vi "SimultaneusWaveformStart.vi"(5 "Ch5Start":bool, 6 "Ch6Start":bool, 7 "Ch4Start":bool, 8 "Ch3Start":bool, 9 "Ch2Start":bool, 10 "Ch1Start":bool, 11 "Handle":u32) -> (3 "FT_Status":u32(ring) items=["FT_OK", "FT_INVALID_HANDLE", "FT_DEVICE_NOT_FOUND", "FT_DEVICE_NOT_OPENED", "FT_IO_ERROR", "FT_INSUFFICIENT_RESOURCES", "FT_INVALID_PARAMETER", "FT_INVALID_BAUD_RATE", "FT_DEVICE_NOT_OPENED_FOR_ERASE", "FT_DEVICE_NOT_OPENED_FOR_WRITE", "FT_FAILED_TO_WRITE_DEVICE", "FT_EEPROM_READ_FAILED", "FT_EEPROM_WRITE_FAILED", "FT_EEPROM_ERASE_FAILED", "FT_EEPROM_NOT_PRESENT", "FT_EEPROM_NOT_PROGRAMMED", "FT_INVALID_ARGS", "FT_NOT_SUPPORTED", "FT_OTHER_ERROR"])   [LabVIEW 2013]
panel:
  out "Bytes Written":u32
  out "Start Array":u8[](array[numeric])
  out "Enable Array":u8[](array[numeric])
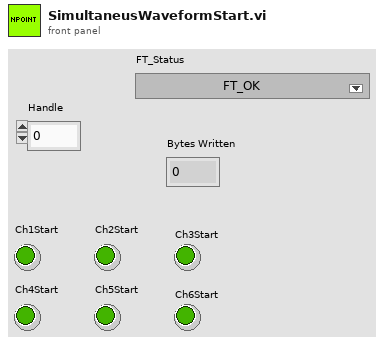
[diagram p1: front panel]
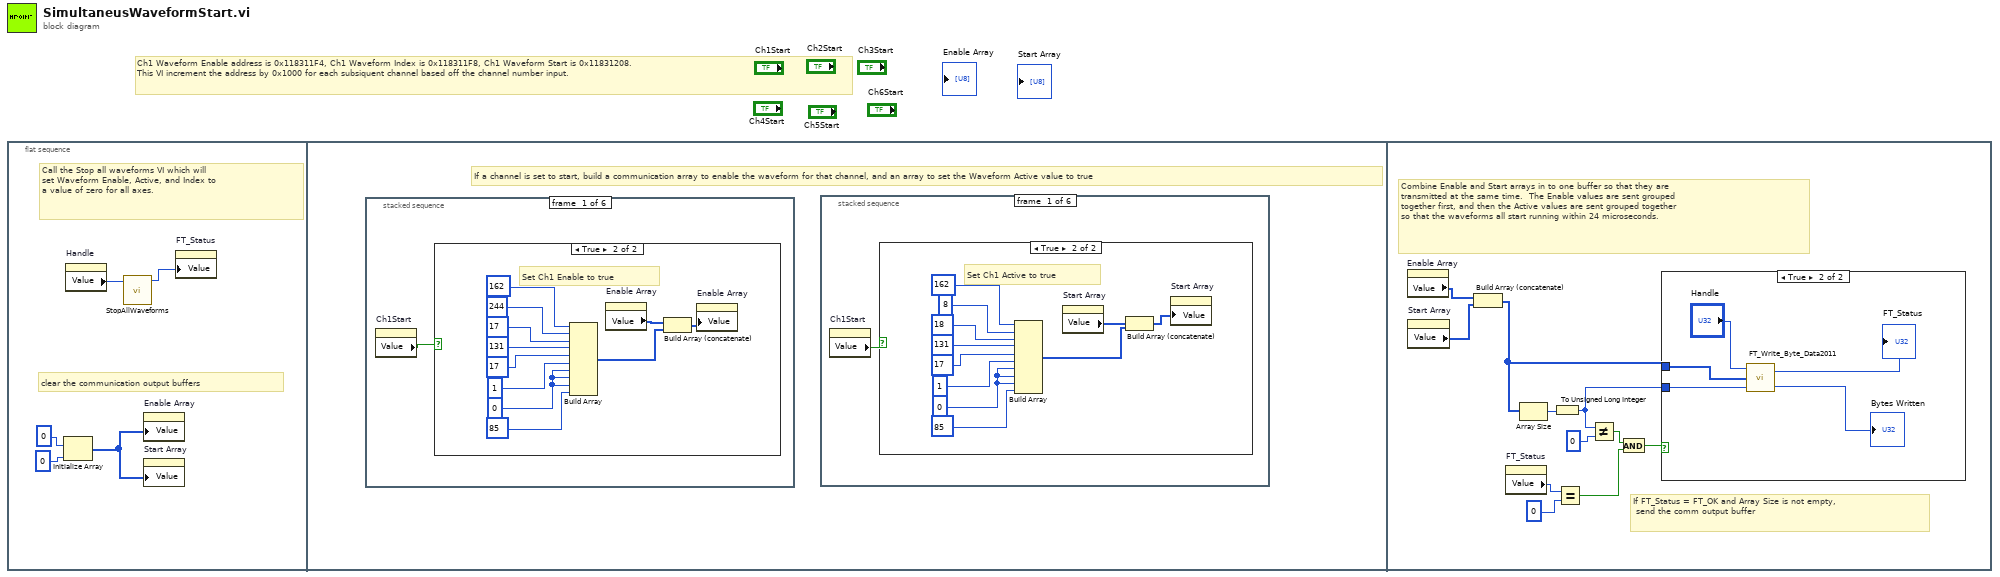
[diagram p0: block diagram]
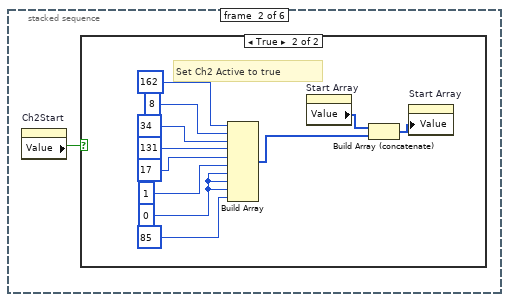
[diagram p3: hidden frame]
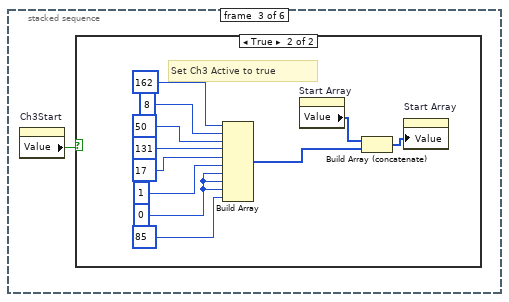
[diagram p5: hidden frame]
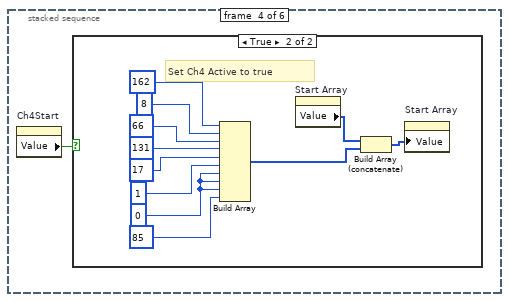
[diagram p7: hidden frame]
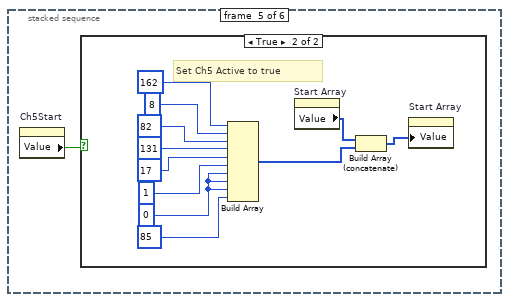
[diagram p9: hidden frame]
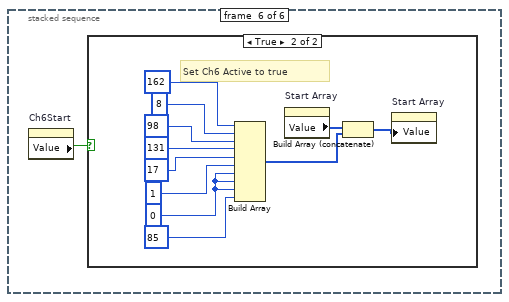
[diagram p11: hidden frame]
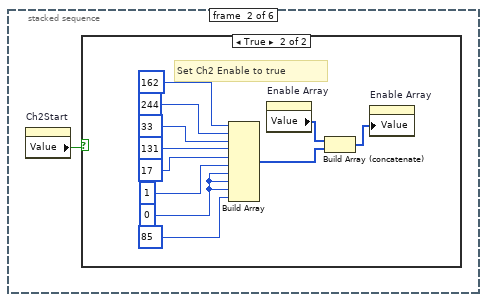
[diagram p14: hidden frame]
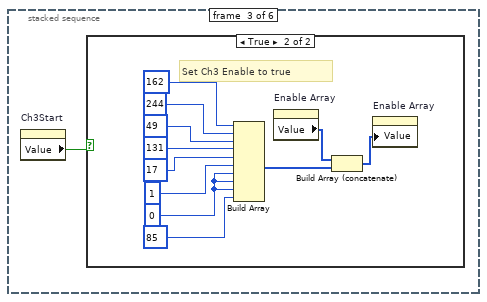
[diagram p16: hidden frame]
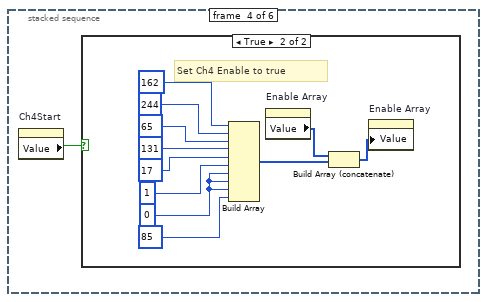
[diagram p18: hidden frame]
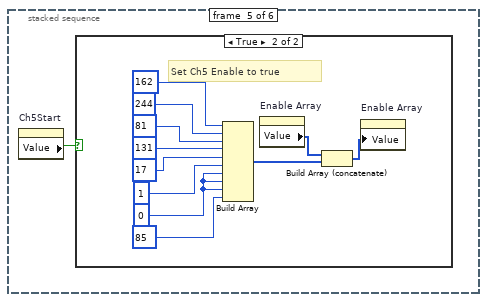
[diagram p20: hidden frame]
diagram:
  # "Ch1 Waveform Enable address is 0x118311F4, Ch1 Waveform Index is 0x118311F8, Ch1 Waveform Start is 0x11831208.\nThis VI increment the address by 0x1000 for each subsiquent channel based off the channel number input."
  n1 = flat-sequence {
    frame #0 {
      # "clear the communication output buffers"
      # "Call the Stop all waveforms VI which will\nset Waveform Enable, Active, and Index to \na value of zero for all axes."
      n2 = Initialize Array(u8 0, 0 ("dimension size")) -> (w1:u8[])
      n3 = property on="Handle" class="DigNum (strict)"() -> ("Value"=w5:u32)  [unwired: 2 in, 2 out]
      n4 = call "StopAllWaveforms.vi"("Handle"=w5) -> ("FT_Status"=w4:u32)  [unwired: 10 in]
      n5 = property on="Enable Array" class="Arr (strict)"("Value"=w1) -> ()  [unwired: 2 in, 2 out]
      n6 = property on="Start Array" class="Arr (strict)"("Value"=w1) -> ()  [unwired: 2 in, 2 out]
      n7 = property on="FT_Status" class="Ring (strict)"("Value"=w4) -> ()  [unwired: 2 in, 2 out]
    }
    frame #1 {
      # "If a channel is set to start, build a communication array to enable the waveform for that channel, and an array to set the Waveform Active value to true"
      n8 = stacked-sequence {
        frame #0 {
          n9 = property on="Ch1Start" class="Bool (strict)"() -> ("Value"=w78:bool)  [unwired: 2 in, 2 out]
          n10 = case shown="True" w78 {
            frame False {
            }
            frame True {
              w83 = u8 0 ("element")
              # "Set Ch1 Enable to true"
              n11 = Build Array(u8 162 ("element"), u8 244 ("element"), u8 17 ("element"), u8 131 ("element"), u8 17 ("element"), u8 1 ("element"), w83, w83, w83, u8 85 ("element")) -> (w80:u8[])
              n12 = property on="Enable Array" class="Arr (strict)"() -> ("Value"=w81:u8[])  [unwired: 2 in, 2 out]
              n13 = Build Array (concatenate)(w81, w80) -> (w79:u8[])
              n14 = property on="Enable Array" class="Arr (strict)"("Value"=w79) -> ()  [unwired: 2 in, 2 out]
            }
          }
        }
        frame #1 {
          n15 = property on="Ch2Start" class="Bool (strict)"() -> ("Value"=w90:bool)  [unwired: 2 in, 2 out]
          n16 = case shown="True" w90 {
            frame False {
            }
            frame True {
              w95 = u8 0 ("element")
              # "Set Ch2 Enable to true"
              n17 = Build Array(u8 162 ("element"), u8 244 ("element"), u8 33 ("element"), u8 131 ("element"), u8 17 ("element"), u8 1 ("element"), w95, w95, w95, u8 85 ("element")) -> (w92:u8[])
              n18 = property on="Enable Array" class="Arr (strict)"() -> ("Value"=w93:u8[])  [unwired: 2 in, 2 out]
              n19 = Build Array (concatenate)(w93, w92) -> (w91:u8[])
              n20 = property on="Enable Array" class="Arr (strict)"("Value"=w91) -> ()  [unwired: 2 in, 2 out]
            }
          }
        }
        frame #2 {
          n21 = property on="Ch3Start" class="Bool (strict)"() -> ("Value"=w102:bool)  [unwired: 2 in, 2 out]
          n22 = case shown="True" w102 {
            frame False {
            }
            frame True {
              w107 = u8 0 ("element")
              # "Set Ch3 Enable to true"
              n23 = Build Array(u8 162 ("element"), u8 244 ("element"), u8 49 ("element"), u8 131 ("element"), u8 17 ("element"), u8 1 ("element"), w107, w107, w107, u8 85 ("element")) -> (w104:u8[])
              n24 = property on="Enable Array" class="Arr (strict)"() -> ("Value"=w105:u8[])  [unwired: 2 in, 2 out]
              n25 = Build Array (concatenate)(w105, w104) -> (w103:u8[])
              n26 = property on="Enable Array" class="Arr (strict)"("Value"=w103) -> ()  [unwired: 2 in, 2 out]
            }
          }
        }
        frame #3 {
          n27 = property on="Ch4Start" class="Bool (strict)"() -> ("Value"=w114:bool)  [unwired: 2 in, 2 out]
          n28 = case shown="True" w114 {
            frame False {
            }
            frame True {
              w119 = u8 0 ("element")
              # "Set Ch4 Enable to true"
              n29 = Build Array(u8 162 ("element"), u8 244 ("element"), u8 65 ("element"), u8 131 ("element"), u8 17 ("element"), u8 1 ("element"), w119, w119, w119, u8 85 ("element")) -> (w116:u8[])
              n30 = property on="Enable Array" class="Arr (strict)"() -> ("Value"=w117:u8[])  [unwired: 2 in, 2 out]
              n31 = Build Array (concatenate)(w117, w116) -> (w115:u8[])
              n32 = property on="Enable Array" class="Arr (strict)"("Value"=w115) -> ()  [unwired: 2 in, 2 out]
            }
          }
        }
        frame #4 {
          n33 = property on="Ch5Start" class="Bool (strict)"() -> ("Value"=w126:bool)  [unwired: 2 in, 2 out]
          n34 = case shown="True" w126 {
            frame False {
            }
            frame True {
              w131 = u8 0 ("element")
              # "Set Ch5 Enable to true"
              n35 = Build Array(u8 162 ("element"), u8 244 ("element"), u8 81 ("element"), u8 131 ("element"), u8 17 ("element"), u8 1 ("element"), w131, w131, w131, u8 85 ("element")) -> (w128:u8[])
              n36 = property on="Enable Array" class="Arr (strict)"() -> ("Value"=w129:u8[])  [unwired: 2 in, 2 out]
              n37 = Build Array (concatenate)(w129, w128) -> (w127:u8[])
              n38 = property on="Enable Array" class="Arr (strict)"("Value"=w127) -> ()  [unwired: 2 in, 2 out]
            }
          }
        }
        frame #5 {
          n39 = property on="Ch6Start" class="Bool (strict)"() -> ("Value"=w138:bool)  [unwired: 2 in, 2 out]
          n40 = case shown="True" w138 {
            frame False {
            }
            frame True {
              w143 = u8 0 ("element")
              # "Set Ch6 Enable to true"
              n41 = Build Array(u8 162 ("element"), u8 244 ("element"), u8 97 ("element"), u8 131 ("element"), u8 17 ("element"), u8 1 ("element"), w143, w143, w143, u8 85 ("element")) -> (w140:u8[])
              n42 = property on="Enable Array" class="Arr (strict)"() -> ("Value"=w141:u8[])  [unwired: 2 in, 2 out]
              n43 = Build Array (concatenate)(w141, w140) -> (w139:u8[])
              n44 = property on="Enable Array" class="Arr (strict)"("Value"=w139) -> ()  [unwired: 2 in, 2 out]
            }
          }
        }
      }
      n45 = stacked-sequence {
        frame #0 {
          n46 = property on="Ch1Start" class="Bool (strict)"() -> ("Value"=w6:bool)  [unwired: 2 in, 2 out]
          n47 = case shown="True" w6 {
            frame False {
            }
            frame True {
              w11 = u8 0 ("element")
              # "Set Ch1 Active to true"
              n48 = Build Array(u8 162 ("element"), u8 8 ("element"), u8 18 ("element"), u8 131 ("element"), u8 17 ("element"), u8 1 ("element"), w11, w11, w11, u8 85 ("element")) -> (w8:u8[])
              n49 = property on="Start Array" class="Arr (strict)"() -> ("Value"=w9:u8[])  [unwired: 2 in, 2 out]
              n50 = Build Array (concatenate)(w9, w8) -> (w7:u8[])
              n51 = property on="Start Array" class="Arr (strict)"("Value"=w7) -> ()  [unwired: 2 in, 2 out]
            }
          }
        }
        frame #1 {
          n52 = property on="Ch2Start" class="Bool (strict)"() -> ("Value"=w18:bool)  [unwired: 2 in, 2 out]
          n53 = case shown="True" w18 {
            frame False {
            }
            frame True {
              w23 = u8 0 ("element")
              # "Set Ch2 Active to true"
              n54 = Build Array(u8 162 ("element"), u8 8 ("element"), u8 34 ("element"), u8 131 ("element"), u8 17 ("element"), u8 1 ("element"), w23, w23, w23, u8 85 ("element")) -> (w20:u8[])
              n55 = property on="Start Array" class="Arr (strict)"() -> ("Value"=w21:u8[])  [unwired: 2 in, 2 out]
              n56 = Build Array (concatenate)(w21, w20) -> (w19:u8[])
              n57 = property on="Start Array" class="Arr (strict)"("Value"=w19) -> ()  [unwired: 2 in, 2 out]
            }
          }
        }
        frame #2 {
          n58 = property on="Ch3Start" class="Bool (strict)"() -> ("Value"=w30:bool)  [unwired: 2 in, 2 out]
          n59 = case shown="True" w30 {
            frame False {
            }
            frame True {
              w35 = u8 0 ("element")
              # "Set Ch3 Active to true"
              n60 = Build Array(u8 162 ("element"), u8 8 ("element"), u8 50 ("element"), u8 131 ("element"), u8 17 ("element"), u8 1 ("element"), w35, w35, w35, u8 85 ("element")) -> (w32:u8[])
              n61 = property on="Start Array" class="Arr (strict)"() -> ("Value"=w33:u8[])  [unwired: 2 in, 2 out]
              n62 = Build Array (concatenate)(w33, w32) -> (w31:u8[])
              n63 = property on="Start Array" class="Arr (strict)"("Value"=w31) -> ()  [unwired: 2 in, 2 out]
            }
          }
        }
        frame #3 {
          n64 = property on="Ch4Start" class="Bool (strict)"() -> ("Value"=w42:bool)  [unwired: 2 in, 2 out]
          n65 = case shown="True" w42 {
            frame False {
            }
            frame True {
              w47 = u8 0 ("element")
              # "Set Ch4 Active to true"
              n66 = Build Array(u8 162 ("element"), u8 8 ("element"), u8 66 ("element"), u8 131 ("element"), u8 17 ("element"), u8 1 ("element"), w47, w47, w47, u8 85 ("element")) -> (w44:u8[])
              n67 = property on="Start Array" class="Arr (strict)"() -> ("Value"=w45:u8[])  [unwired: 2 in, 2 out]
              n68 = Build Array (concatenate)(w45, w44) -> (w43:u8[])
              n69 = property on="Start Array" class="Arr (strict)"("Value"=w43) -> ()  [unwired: 2 in, 2 out]
            }
          }
        }
        frame #4 {
          n70 = property on="Ch5Start" class="Bool (strict)"() -> ("Value"=w54:bool)  [unwired: 2 in, 2 out]
          n71 = case shown="True" w54 {
            frame False {
            }
            frame True {
              w59 = u8 0 ("element")
              # "Set Ch5 Active to true"
              n72 = Build Array(u8 162 ("element"), u8 8 ("element"), u8 82 ("element"), u8 131 ("element"), u8 17 ("element"), u8 1 ("element"), w59, w59, w59, u8 85 ("element")) -> (w56:u8[])
              n73 = property on="Start Array" class="Arr (strict)"() -> ("Value"=w57:u8[])  [unwired: 2 in, 2 out]
              n74 = Build Array (concatenate)(w57, w56) -> (w55:u8[])
              n75 = property on="Start Array" class="Arr (strict)"("Value"=w55) -> ()  [unwired: 2 in, 2 out]
            }
          }
        }
        frame #5 {
          n76 = property on="Ch6Start" class="Bool (strict)"() -> ("Value"=w66:bool)  [unwired: 2 in, 2 out]
          n77 = case shown="True" w66 {
            frame False {
            }
            frame True {
              w71 = u8 0 ("element")
              # "Set Ch6 Active to true"
              n78 = Build Array(u8 162 ("element"), u8 8 ("element"), u8 98 ("element"), u8 131 ("element"), u8 17 ("element"), u8 1 ("element"), w71, w71, w71, u8 85 ("element")) -> (w68:u8[])
              n79 = property on="Start Array" class="Arr (strict)"() -> ("Value"=w69:u8[])  [unwired: 2 in, 2 out]
              n80 = Build Array (concatenate)(w69, w68) -> (w67:u8[])
              n81 = property on="Start Array" class="Arr (strict)"("Value"=w67) -> ()  [unwired: 2 in, 2 out]
            }
          }
        }
      }
    }
    frame #2 {
      # "If FT_Status = FT_OK and Array Size is not empty,\n send the comm output buffer"
      # "Combine Enable and Start arrays in to one buffer so that they are\ntransmitted at the same time.  The Enable values are sent grouped \ntogether first, and then the Active values are sent grouped together\nso that the waveforms all start running within 24 microseconds."
      n82 = property on="Enable Array" class="Arr (strict)"() -> ("Value"=w159:u8[])  [unwired: 2 in, 2 out]
      n83 = property on="Start Array" class="Arr (strict)"() -> ("Value"=w158:u8[])  [unwired: 2 in, 2 out]
      n84 = Build Array (concatenate)(w159, w158) -> (w157:u8[])
      n85 = property on="FT_Status" class="Ring (strict)"() -> ("Value"=w156:u32)  [unwired: 2 in, 2 out]
      n86 = Array Size(array=w157) -> (size(s)=w160:i32)
      n87 = To Unsigned Long Integer(number=w160) -> (unsigned 32bit integer=w154:u32)
      n88 = Equal?(x=w156, y=u32 0) -> (x = y?=w151:bool)
      n89 = Not Equal?(x=w154, y=u32 0) -> (x != y?=w152:bool)
      n90 = And(x=w152, y=w151) -> (x .and. y?=w150:bool)
      n91 = case shown="True" w150 {
        tunnel: w154 -> [_ w165]
        tunnel: w157 -> [_ w161]
        frame False {
        }
        frame True {
          n92 = call "FT_Write_Byte_Data2011.vi"("Bytes To Write"=w165, "Buffer"=w161, "Handle"="Handle") -> ("Bytes Written"=→"Bytes Written":u32, "FT_Status"=→"FT_Status":u32)
        }
      }
    }
  }
